vi "Compiled.Get Data Settings.vi"(6 "Cluster":refnum<k21>, 8 "error in (no error)":errorcluster, 9 "Node.Settings":T3 {"Name" format="%.0x"}, 10 "Node Ref in":T1 format="%.0x", 11 "Addon Ref In":T1 format="%.0x") -> (0 "error out":errorcluster, 1 "Node Data Refs":T4 {"Outgoing"."Trigger.Refs"."Data Reference" format="%.0x"; "Outgoing"."Disable.Refs"."Data Reference" format="%.0x"; "Outgoing"."Data.Refs"."Data Reference" format="%.0x"; "Incoming"."Timing.Refs"."Data Reference" format="%.0x"; "Incoming"."Data.Refs"."Data Reference" format="%.0x"}, 2 "Node Ref out":T1 format="%.0x", 3 "Addon Ref out":T1 format="%.0x", 4 "Async Refs":T2(array[cluster]) {"VS Refs" format="%.0x"})   [LabVIEW 2023, in "J1939 Addon System Explorer.lvlib"]
uses:
  J1939 Addon System Explorer.lvlib
  Addon Shared/Types/Device Settings.ctl
  Addon Shared/Types/Incoming Settings.ctl
  Addon Shared/Types/Incoming Frame Settings.ctl
  <vilib>/NI VeriStand/Custom Device API/Block Data Reference.ctl
  <vilib>/NI VeriStand/Custom Device API/Data Reference.ctl
  Addon Shared/Types/Outgoing Settings.ctl
  Addon Shared/Types/Outgoing Frame Settings.ctl
  Addon Shared/Types/Outgoing Event Trigger Types.ctl
  SubModules/Frame-Protection-Support/Source/Shared/Types/Exported Frame Settings.ctl
  SubModules/Frame-Protection-Support/Source/Shared/Types/Exported Frame Type.ctl
  SubModules/Frame-Protection-Support/Source/Shared/Types/Exported Protection Settings.ctl
  SubModules/Frame-Protection-Support/Source/Shared/Types/Protection Type.ctl
  SubModules/Frame-Protection-Support/Source/Shared/Types/XNET Signal Configuration.ctl
  SubModules/Frame-Protection-Support/Source/Shared/Types/Exported Counter Settings.ctl
  SubModules/Frame-Protection-Support/Source/Shared/Types/Exported Event Trigger Type.ctl
  <vilib>/NI VeriStand/Custom Device API/Custom Device Item Ref.ctl
  Addon Shared/Types/Monitor Settings.ctl
  SubModules/Frame-Protection-Support/Source/System Explorer/Types/Export Frame GUIDs List.ctl
  Types/Compiled Refs.ctl
  <vilib>/NI VeriStand/Custom Device API/Data Access Type.ctl
  SubModules/Frame-Protection-Support/Source/System Explorer/Types/Export Frames List and Type.ctl
  SubModules/Frame-Protection-Support/Source/System Explorer/Types/Exported Frame Settings.ctl
  Addon Shared/SubVIs/Constants.vi
  <vilib>/NI VeriStand/Custom Device Tools/Custom Device Utility Library/NI VeriStand - Search for Item by GUID.vi
  <vilib>/NI VeriStand/Custom Device Tools/Custom Device Utility Library/Custom Device Utility Library.lvlib
  Addon Shared/J1939 Addon Shared.lvlib
  <vilib>/NI VeriStand/Custom Device API/Custom Device API.lvlib
  SubModules/Frame-Protection-Support/Source/Shared/Protection and Counter Support Shared.lvlib
  SubModules/Frame-Protection-Support/Source/System Explorer/Protection and Counter Support System Explorer.lvlib
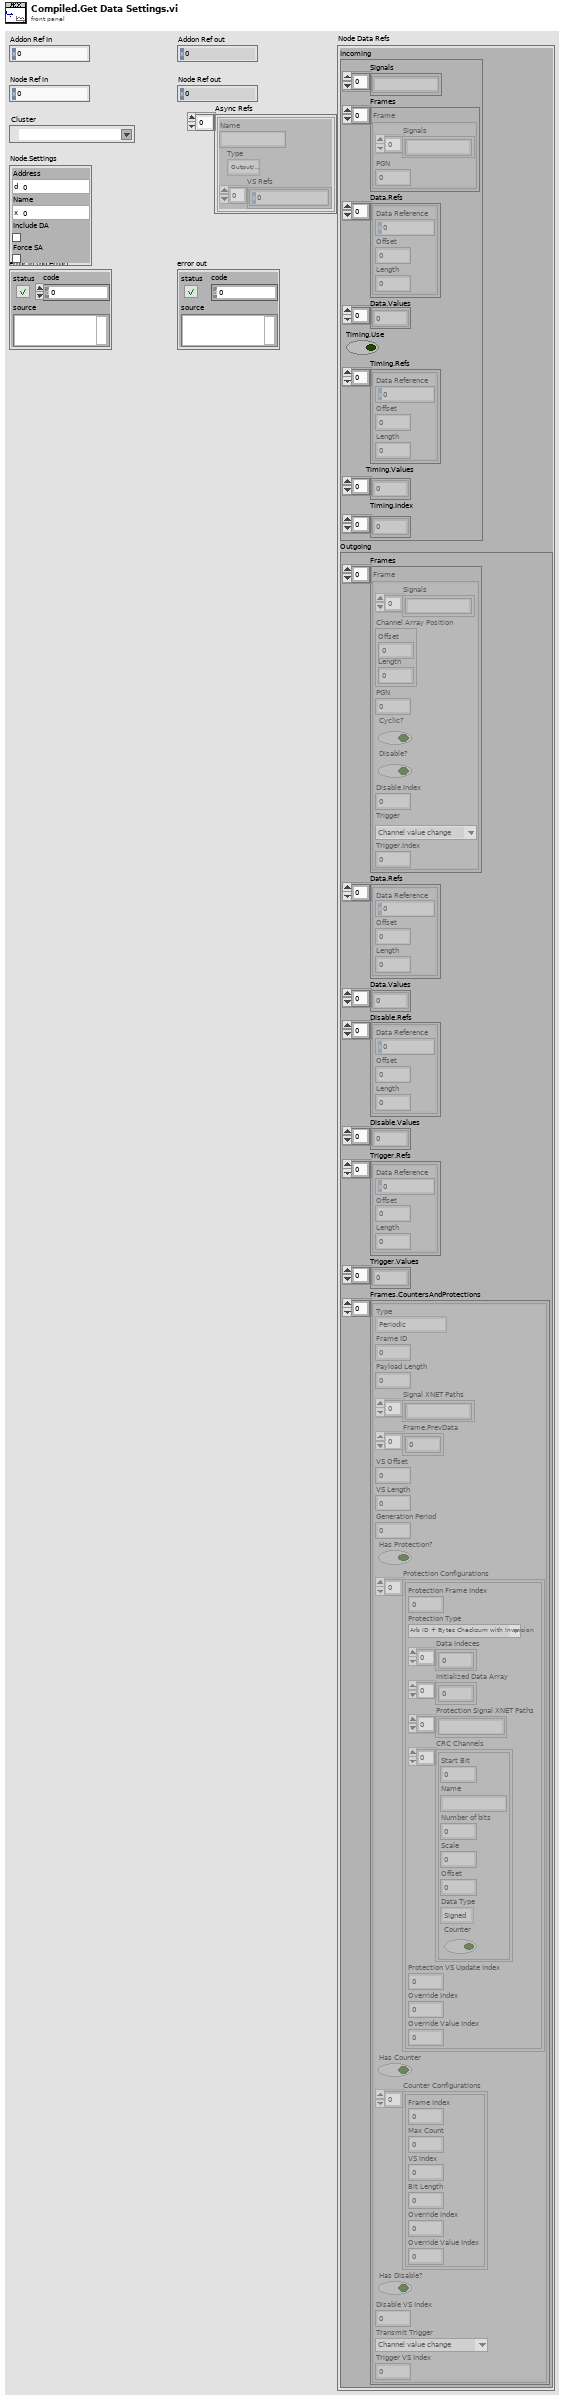
[diagram p1: front panel]
types:
  T1 = typedef "Custom Device API.lvlib/Custom Device Item Ref.ctl" = u64
  T2 = cluster{"Name":string, "Type":enum16{"Output/Write", "Input/Read", "Input/ReadWrite"}, "VS Refs":T1[]}[]
  T3 = typedef "J1939 Addon Shared.lvlib/Monitor Settings.ctl" = cluster{"Address":u8, "Name":u64, "Include DA":bool, "Force SA":bool}
  T4 = typedef "J1939 Addon Shared.lvlib/Device Settings.ctl" = cluster{"Incoming":T5, "Outgoing":T9}
  T5 = typedef "J1939 Addon Shared.lvlib/Incoming Settings.ctl" = cluster{"Signals":string[], "Frames":T6[], "Data.Refs":T7[], "Data.Values":dbl[], "Timing.Use":bool, "Timing.Refs":T7[], "Timing.Values":dbl[], "Timing.Index":i32[]}
  T6 = typedef "J1939 Addon Shared.lvlib/Incoming Frame Settings.ctl" = cluster{"Signals":string[], "PGN":u32}
  T7 = typedef "Custom Device API.lvlib/Block Data Reference.ctl" = cluster{"Data Reference":T8, "Offset":u64, "Length":u64}
  T8 = typedef "Custom Device API.lvlib/Data Reference.ctl" = i32
  T9 = typedef "J1939 Addon Shared.lvlib/Outgoing Settings.ctl" = cluster{"Frames":T10[], "Data.Refs":T7[], "Data.Values":dbl[], "Disable.Refs":T7[], "Disable.Values":dbl[], "Trigger.Refs":T7[], "Trigger.Values":dbl[], "Frames.CountersAndProtections":T12[]}
  T10 = typedef "J1939 Addon Shared.lvlib/Outgoing Frame Settings.ctl" = cluster{"Signals":string[], "Channel Array Position":cluster{"Offset":u32, "Length":u32}, "PGN":u32, "Cyclic?":bool, "Disable?":bool, "Disable.Index":i32, "Trigger":T11, "Trigger.Index":i32}
  T11 = typedef "J1939 Addon Shared.lvlib/Outgoing Event Trigger Types.ctl" = enum16{"Channel value change", "Trigger channel (not zero)", "Channel value change or trigger channel (not zero)", "Trigger channel (any value change)", "Channel value change or trigger channel (any value change)"}
  T12 = typedef "Protection and Counter Support Shared.lvlib/Exported Frame Settings.ctl" = cluster{"Type":T13, "Frame ID":u32, "Payload Length":u32, "Signal XNET Paths":string[], "Frame.PrevData":dbl[], "VS Offset":i32, "VS Length":i32, "Generation Period":u32, "Has Protection?":bool, "Protection Configurations":T14[], "Has Counter":bool, "Counter Configurations":T17[], "Has Disable?":bool, "Disable VS Index":i32, "Transmit Trigger":T18, "Trigger VS Index":i32}
  T13 = typedef "Protection and Counter Support Shared.lvlib/Exported Frame Type.ctl" = enum16{"Periodic", "Event", "Periodic/Event"}
  T14 = typedef "Protection and Counter Support Shared.lvlib/Exported Protection Settings.ctl" = cluster{"Protection Frame Index":i32, "Protection Type":T15, "Data Indeces":i32[], "Initialized Data Array":dbl[], "Protection Signal XNET Paths":string[], "CRC Channels":T16[], "Protection VS Update Index":i32, "Override Index":i32, "Override Value Index":i32}
  T15 = typedef "Protection and Counter Support Shared.lvlib/Protection Type.ctl" = enum16{"Arb ID + Bytes Checksum with Inversion", "Arb ID + Bytes CRC with Inversion", "Reversed Raw Signal Checksum with Inversion", "Concatenated Two's Compliment"}
  T16 = typedef "Protection and Counter Support Shared.lvlib/XNET Signal Configuration.ctl" = cluster{"Start Bit":i32, "Name":string, "Number of bits":i32, "Scale":dbl, "Offset":dbl, "Data Type":u32, "Counter":bool}
  T17 = typedef "Protection and Counter Support Shared.lvlib/Exported Counter Settings.ctl" = cluster{"Frame Index":i32, "Max Count":dbl, "VS Index":i32, "Bit Length":i64, "Override Index":i32, "Override Value Index":i32}
  T18 = typedef "Protection and Counter Support Shared.lvlib/Exported Event Trigger Type.ctl" = enum16{"Channel value change", "Trigger channel (not zero)", "Channel value change or trigger channel (not zero)", "Trigger channel (any value change)", "Channel value change or trigger channel (any value change)"}
  T19 = cluster{"Name":string, "Type":enum16{"Output/Write", "Input/Read", "Input/ReadWrite"}, "VS Refs":T1[]}
  T20 = typedef "Protection and Counter Support System Explorer.lvlib/Export Frame GUIDs List.ctl" = cluster{"Signal Page GUID":string, "Rolling Counter Value GUID":string, "Protection Value GUID":string}
  T21 = typedef "J1939 Addon System Explorer.lvlib/Compiled Refs.ctl" = cluster{"VS Refs":T1[], "Disable Refs":T1[], "Trigger Refs":T1[]}
  T22 = typedef "Custom Device API.lvlib/Data Access Type.ctl" = enum16{"Read", "Write"}
  T23 = typedef "Protection and Counter Support System Explorer.lvlib/Export Frames List and Type.ctl" = cluster{"Type":T13, "Frame Refs":T1[], "Frame Settings":T24[]}
  T24 = typedef "Protection and Counter Support System Explorer.lvlib/Exported Frame Settings.ctl" = cluster{"ID":u32, "Disable Transmission":bool, "Disable Transmission Ref":T1, "Transmit Trigger":T18, "Transmit Trigger Ref":T1}
  T25 = typedef "J1939 Addon Shared.lvlib/Frame.Settings.ctl" = cluster{"ID":u32, "Disable Transmission":bool, "Disable Transmission Ref":T1, "Transmit Trigger":T11, "Transmit Trigger Ref":T1}
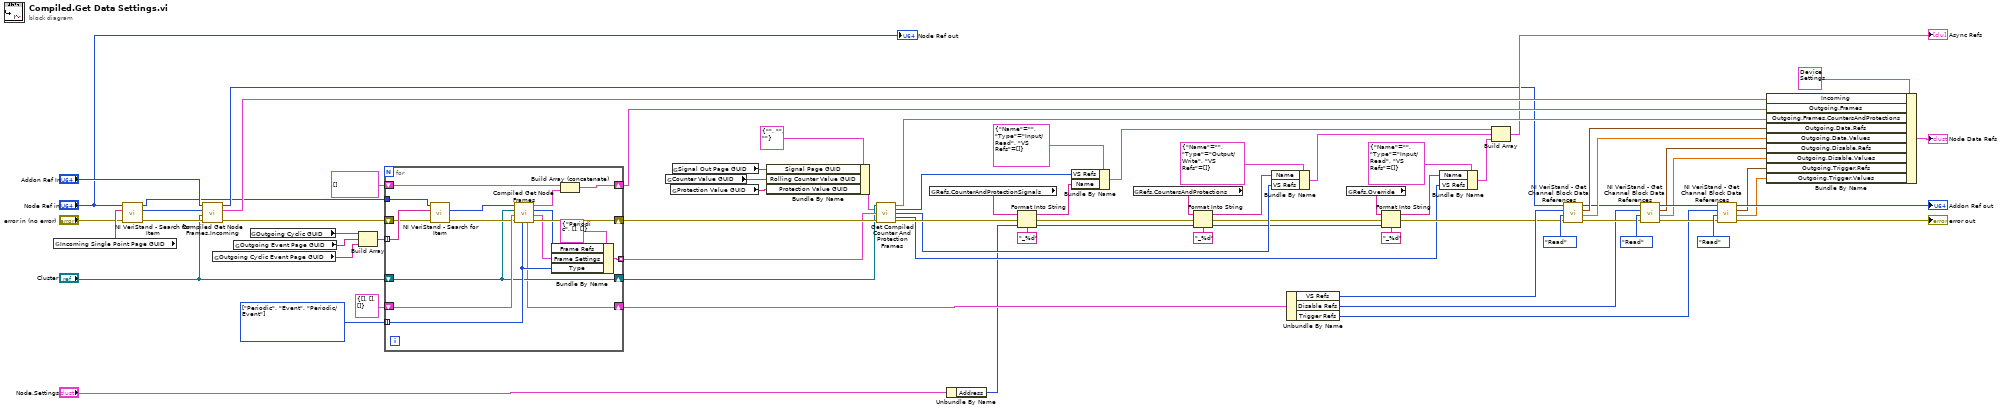
[diagram p0: block diagram]
diagram:
  w44 = T13[] [enum."Periodic", enum."Event", enum."Periodic/Event"] items=["Periodic", "Event", "Periodic/Event"]
  n1 = global read "Constants.vi" "Incoming Single Point Page GUID"() -> (w69:string)
  n2 = call-poly <vilib>:"NI VeriStand - Search for Item.vi"("error in"="error in (no error)", "Item GUID"=w69, "Section Ref in"="Node Ref in") -> ("error out"=w66:errorcluster, "Item Ref"=w67:T1, "Section Ref out"=w13:T1)  [unwired: 5 in, 1 out]
  n3 = call "Compiled Get Node Frames.Incoming.vi"("error in (no error)"=w66, "Cluster"="Cluster", "Section Ref in"=w67, "Device Ref in"="Addon Ref In") -> ("error out"=w32:errorcluster, "Incoming.Settings"=w64:T5, "Device Ref out"=w14:T1)  [unwired: 5 in]
  n4 = global read "Constants.vi" "Outgoing Cyclic Event Page GUID"() -> (w46:string)
  n5 = global read "Constants.vi" "Outgoing Event Page GUID"() -> (w47:string)
  n6 = global read "Constants.vi" "Outgoing Cyclic GUID"() -> (w48:string)
  n7 = Build Array(w48, w47, w46) -> (w45:string[])
  n8 = for {
    tunnel: w45 -> [w91] mode=indexing
    tunnel: w44 -> [w82] mode=indexing
    shift-right: [w76] -> w33
    shift-left: T21 {"VS Refs"=[], "Disable Refs"=[], "Trigger Refs"=[]} ("Refs out") -> [w89]
    shift-right: [w88] -> w41
    shift-left: w32 -> [w87]
    shift-right: [w85] -> w35
    shift-left: T10[] [] -> [w84]
    tunnel: [w80] -> w40 mode=indexing
    shift-right: [w77] -> w31
    shift-left: "Cluster" -> [w77]
    tunnel: w13 -> [w79]
    n9 = call-poly <vilib>:"NI VeriStand - Search for Item.vi"("error in"=w87, "Item GUID"=w91, "Section Ref in"=w79) -> ("error out"=w78:errorcluster, "Item Ref"=w90:T1)  [unwired: 5 in, 2 out]
    n10 = call "Compiled Get Node Frames.vi"("Type"=w82, "error in (no error)"=w78, "Refs in"=w89, "Cluster"=w77, "Section Ref in"=w90) -> ("error out"=w88:errorcluster, "Counter and Protection Frames Properties"=w75:T25[], "Counter and Protection Frames"=w81:T1[], "Standard Frames"=w86:T10[], "Refs out"=w76:T21)  [unwired: 2 in]
    n11 = Bundle By Name(cluster=T23 {"Type"=enum."Periodic", "Frame Refs"=[], "Frame Settings"=[]}, "Frame Refs"=w81, "Frame Settings"=w75, "Type"=w82) -> (w80:T23)
    n12 = Build Array (concatenate)(w84, w86) -> (w85:T10[])
  }
  n13 = global read "Constants.vi" "Counter Value GUID"() -> (w37:string)
  n14 = global read "Constants.vi" "Protection Value GUID"() -> (w36:string)
  n15 = global read "Constants.vi" "Signal Out Page GUID"() -> (w38:string)
  n16 = Bundle By Name(cluster=T20 {"Signal Page GUID"="", "Rolling Counter Value GUID"="", "Protection Value GUID"=""} ("GUIDs"), "Signal Page GUID"=w38, "Rolling Counter Value GUID"=w37, "Protection Value GUID"=w36) -> (w10:T20)
  n17 = call "Get Compiled Counter And Protection Frames.vi"("XNET Cluster"=w31, "GUIDs"=w10, "Frames per type"=w40, "error in (no error)"=w41) -> ("Frames"=w34:T12[], "Signals Refs"=w21:T1[], "Counters and Protection Refs"=w18:T1[], "Override Refs"=w2:T1[], "error out"=w24:errorcluster)  [unwired: 7 in]
  n18 = global read "Constants.vi" "Refs.CounterAndProtectionSignals"() -> (w28:string)
  n19 = Unbundle By Name("Node.Settings") -> ("Address"=w1:u8)
  n20 = Format Into String(format string="_%d", initial string=w28, error in=w24, w1) -> (resulting string=w22:string, error out=w26:errorcluster)
  n21 = Bundle By Name(cluster=T19 {"Name"="", "Type"=enum."Input/Read", "VS Refs"=[]} ("Group"), "VS Refs"=w21, "Name"=w22) -> (w17:T19)
  n22 = global read "Constants.vi" "Refs.CountersAndProtections"() -> (w25:string)
  n23 = Format Into String(format string="_%d", initial string=w25, error in=w26, w1) -> (resulting string=w19:string, error out=w4:errorcluster)
  n24 = Bundle By Name(cluster=T19 {"Name"="", "Type"=enum."Output/Write", "VS Refs"=[]} ("Group"), "Name"=w19, "VS Refs"=w18) -> (w16:T19)
  n25 = Unbundle By Name(w33) -> ("VS Refs"=w55:T1[], "Disable Refs"=w54:T1[], "Trigger Refs"=w53:T1[])
  n26 = global read "Constants.vi" "Refs.Override"() -> (w7:string)
  n27 = Format Into String(format string="_%d", initial string=w7, error in=w4, w1) -> (resulting string=w9:string, error out=w3:errorcluster)
  n28 = Bundle By Name(cluster=T19 {"Name"="", "Type"=enum."Input/Read", "VS Refs"=[]} ("Group"), "Name"=w9, "VS Refs"=w2) -> (w5:T19)
  n29 = Build Array(w17, w16, w5) -> (→"Async Refs":T2)
  n30 = call <vilib>:"NI VeriStand - Get Channel Block Data References.vi"("error in (no error)"=w3, "Access"=Data_Access_Type."Read", "Channel Refs"=w55, "Device Ref in"=w14) -> ("error out"=w61:errorcluster, "Values Array"=w72:dbl[], "Block Data Refs"=w71:T7[], "Device Ref out"=w57:T1)  [unwired: 4 in]
  n31 = call <vilib>:"NI VeriStand - Get Channel Block Data References.vi"("error in (no error)"=w61, "Access"=Data_Access_Type."Read", "Channel Refs"=w54, "Device Ref in"=w57) -> ("error out"=w60:errorcluster, "Values Array"=w50:dbl[], "Block Data Refs"=w49:T7[], "Device Ref out"=w58:T1)  [unwired: 4 in]
  n32 = call <vilib>:"NI VeriStand - Get Channel Block Data References.vi"("error in (no error)"=w60, "Access"=Data_Access_Type."Read", "Channel Refs"=w53, "Device Ref in"=w58) -> ("error out"=→"error out":errorcluster, "Values Array"=w52:dbl[], "Block Data Refs"=w51:T7[], "Device Ref out"=→"Addon Ref out":T1)  [unwired: 4 in]
  n33 = Bundle By Name(cluster=T4 {"Incoming"={"Signals"=[], "Frames"=[], "Data.Refs"=[], "Data.Values"=[], "Timing.Use"=FALSE, "Timing.Refs"=[], "Timing.Values"=[], "Timing.Index"=[]}, "Outgoing"={"Frames"=[], "Data.Refs"=[], "Data.Values"=[], "Disable.Refs"=[], "Disable.Values"=[], "Trigger.Refs"=[], "Trigger.Values"=[], "Frames.CountersAndProtections"=[]}} ("Data"), "Incoming"=w64, "Outgoing.Frames"=w35, "Outgoing.Frames.CountersAndProtections"=w34, "Outgoing.Data.Refs"=w71, "Outgoing.Data.Values"=w72, "Outgoing.Disable.Refs"=w49, "Outgoing.Disable.Values"=w50, "Outgoing.Trigger.Refs"=w51, "Outgoing.Trigger.Values"=w52) -> (→"Node Data Refs":T4)
  "Node Ref out" <- "Node Ref in"
